vi "Problem 25.vi"() -> ()   [LabVIEW 2013, in "Problem 25.lvlib"]
uses:
  Problem 25.lvlib
panel:
  out "Answer":i32
  out "fib(n)":string
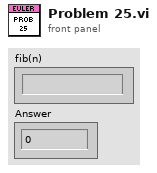
[diagram p1: front panel]
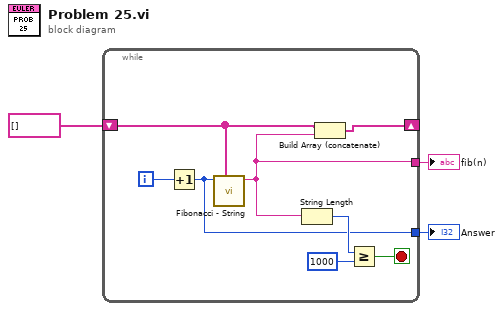
[diagram p0: block diagram]
diagram:
  n1 = while {
    shift-right: [w9] -> _
    shift-left: string[] [] ("Memo") -> [w10]
    tunnel: [w6] -> w2
    tunnel: [w4] -> w1
    i -> [w11]
    stop <- w5 stop-if-true
    n2 = Increment(x=w11) -> (x+1=w4:i32)
    n3 = call "Fibonacci - String.vi"("Memo"=w10, "n"=w4) -> ("fib(n)"=w6:string)  [unwired: 9 in]
    n4 = String Length(string=w6) -> (length=w8:i32)
    n5 = Build Array (concatenate)(w10, w6) -> (w9:string[])
    n6 = Greater Or Equal?(x=w8, y=1000) -> (x >= y?=w5:bool)
  }
  "fib(n)" <- w2
  "Answer" <- w1
